vi "5.1-4.7.1-Act Server.vi"() -> ()   [LabVIEW 2010]
doc: "Creates a named service and listens on the first available port. Whenever a client connects to the service, it responds with a message containing joystick data. The VI can be stopped using the STOP button."
uses:
  6-OCU Neurons/6.0-Super Heart Beat.ctl
  5.7-UDP/5.7 LabVIEW Errors.ctl
  5.0-Global.vi
panel:
  out "Super Heart Beat":T1
  out "error out":errorcluster
  in  "stop":bool
  out "Probably a hello string":string
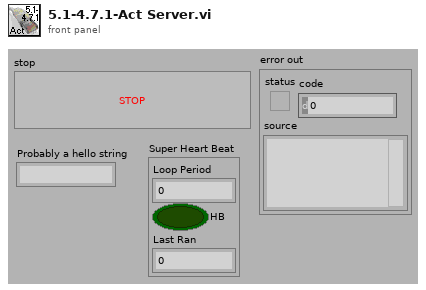
[diagram p1: front panel]
types:
  T1 = typedef "6.0-Super Heart Beat.ctl" = cluster{"Loop Period":u32, "HB":bool, "Last Ran":u32}
  T2 = typedef "4.1-Act Control Typedef.ctl" = cluster{"4.1.0 Data":variant, "Type of Data":T3, "E-Stop":bool, "Restart":bool, "New IP":bool, "Begin":bool, "Time":i32, "Shutdown":bool}
  T3 = typedef "4.1.0-Datatype Typedef.ctl" = enum16{"4.1.0-Empty Data", "4.1.1-Joystick Data", "4.1.2-Behavioral Data"}
  T4 = typedef "5.7 LabVIEW Errors.ctl" = i32
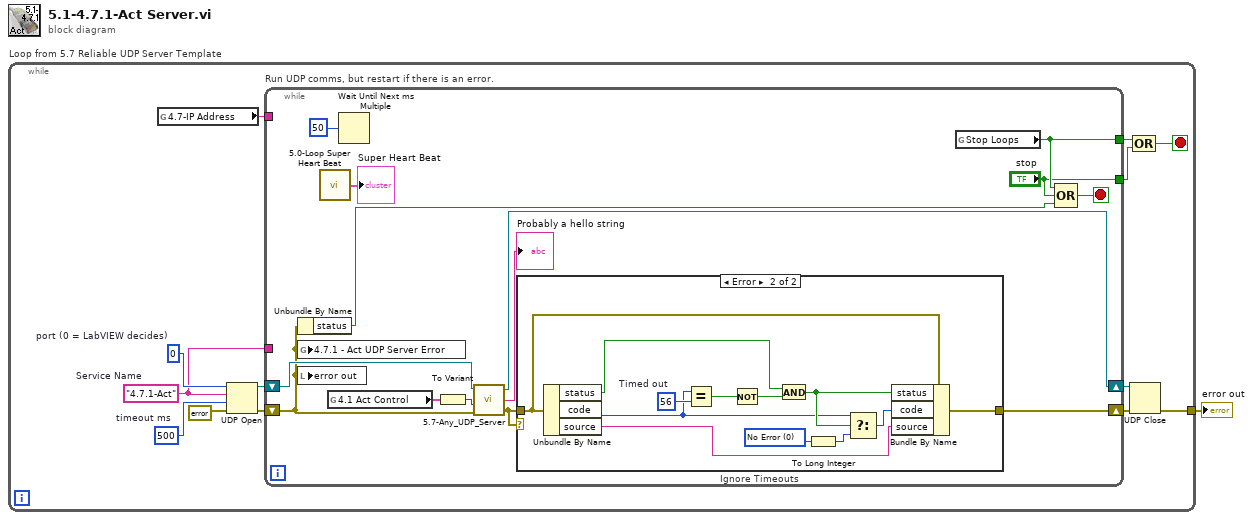
[diagram p0: block diagram]
diagram:
  n1 = while "Loop from 5.7 Reliable UDP Server Template" {
    tunnel: [w2] -> w1
    stop <- w12 stop-if-true
    w5 = 500  # timeout ms
    w7 = u16 0  # port (0 = LabVIEW decides)
    w6 = "4.7.1-Act"  # Service Name
    n2 = global read "5.0-Global.vi" "4.7-IP Address"() -> (w4:string)
    n3 = UDP Open(8:errorcluster {"status"=FALSE, "code"=0, "source"=""} ("error in (no error)"), 9:w5, 10:w6, 11:w7) -> (port=w11:refnum<k16>, 0:w9:errorcluster)  [unwired: 1 in, 1 out]
    n4 = while "Run UDP comms, but restart if there is an error." {
      tunnel: w6 -> [_]
      tunnel: w4 -> [_]
      tunnel: [w26] -> w14
      tunnel: ["stop"] -> w13
      shift-right: [w21] -> w10
      shift-left: w11 -> [w22]
      shift-right: [w23] -> w8
      shift-left: w9 -> [w15]
      stop <- w28 stop-if-true
      n5 = Unbundle By Name(w15) -> ("status"=w24:bool)
      n6 = global write "5.0-Global.vi" "4.7.1 - Act UDP Server Error"(w15) -> ()
      n7 = local write "error out"(w15) -> ()
      n8 = call "5.0-Loop Super Heart Beat.vi"() -> ("Super Heart Beat"=→"Super Heart Beat":T1)
      n9 = global read "5.0-Global.vi" "4.1 Act Control"() -> (w18:T2)
      n10 = Wait Until Next ms Multiple(millisecond multiple=u32 50) -> ()  [unwired: 1 out]
      n11 = To Variant(anything=w18) -> (Variant=w20:variant)
      n12 = call "5.7-Any_UDP_Server.vi"("error In"=w15, "Data in"=w20, "Connection ID"=w22) -> ("warning out"=w16:errorcluster, "data out"=→"Probably a hello string":string, "Connection ID out"=w21:refnum<k16>)  [unwired: 1 in]
      n13 = case "Ignore Timeouts" shown="Error" w16 {
        tunnel: w16 -> [w29 w41]
        tunnel: [w29 w40] -> w23
        frame No Error {
        }
        frame Error {
          w31 = T4 0 items=["No Error", "Argument Error", "Memory Full", "Out of Zone", "End of File", "File Already Open", "Generic File IO Error", "File Not Found", "File Permission Error", "Disk Full", "Duplicate Path", "Too Many Files Open", "Not Enabled", "Resource File Not Found", "Cannot Add Resource", "Resource Not Found", "Image Not Found", "Image Memory Error", "Pen Does Not Exist", "Config Bad Type", "Config Token Not Found", "Config Parse Error", "Config Memory Error", "Bad External Code Format", "Bad External Code Offset", "External Code Not Present", "Null Window", "Destroy Window Mixup", "Null Menu", "Print Aborted", "Bad Print Record", "Print Driver Error", "Windows Error During Print", "Memory Error During Print", "Print Dialog Error", "Generic Print Error", "Invalid Device Refnum", "Device Not Found", "Device Parameter Error", "Device Unit Error", "Can't Open Device", "Device Call Aborted", "Generic Error", "Cancelled By User", "Object ID Too Low", "Object ID Too High", "Object Not In Heap", "Unknown Heap", "Bad DefProc ID", "DefProc Not In Table", "Message Out Of Range", "Null Method", "Unknown Message", "Manager Call Not Supported", "Bad address", "Connection In progress", "Connection timed out", "Connection is already in progress", "Network attribute not supported", "Network error", "Address in use", "System out of memory", "Connection aborted", "Connection refused", "Connection is not connected", "Connection is already connected", "Connection closed", "Initialize error (interapplication manager)", "Bad occurrence", "Wait on unbound occurrence handler", "Occurrence queue overflow", "Bad path", "Semaphore not signaled", "Unrecognized type (interapplication manager)"] ("1st Error to Convert")
          w39 = 56  # Timed out
          n14 = Unbundle By Name(w41) -> ("status"=w36:bool, "code"=w34:i32, "source"=w32:string)
          n15 = Equal?(x=w34, y=w39) -> (x = y?=w38:bool)
          n16 = Not(x=w38) -> (.not. x?=w37:bool)
          n17 = And(x=w36, y=w37) -> (x .and. y?=w35:bool)
          n18 = To Long Integer(number=w31) -> (32bit integer=w30:T4)
          n19 = Select(t=w34, s=w35, f=w30) -> (s? t:f=w33:T4)
          n20 = Bundle By Name(cluster=w41, "status"=w35, "code"=w33, "source"=w32) -> (w40:errorcluster)
        }
      }
      n21 = global read "5.0-Global.vi" "Stop Loops"() -> (w26:bool)
      n22 = Compound Arithmetic op=OR(w26, "stop", w24) -> (w28:bool)
    }
    n23 = UDP Close(connection ID=w10, 8:w8) -> (error out=w2:errorcluster)  [unwired: 1 out]
    n24 = Compound Arithmetic op=OR(w14, w13) -> (w12:bool)
  }
  "error out" <- w1
